vi "get_spiral_parameters.vi"(8 "error in (no error)":errorcluster, 11 "ImageAssemblerRK110612Spiral in":refnum<class "ImageAssemblerRK110612Spiral.lvclass">) -> (0 "error out":errorcluster, 2 "Fiber spiral parameters":T1={"Fiber Frequency"=2200, "Imaging Periods"=100, "Settling Periods"=50, "Resting Periods"=30, "Amplitude X"=0.5, "Amplitude Y"=0.5, "Phase difference"=90.0, "Initial Amplitude X"=0.0, "Initial Amplitude Y"=0.0} {"Initial Amplitude Y" min=0.0 max=3.0 step=0.1; "Initial Amplitude X" min=0.0 max=3.0 step=0.1; "Phase difference" min=0.0 max=360.0 step=5.0; "Amplitude Y" min=0.0 max=3.0 step=0.1; "Amplitude X" min=0.0 max=3.0 step=0.1}, 3 "ImageAssemblerRK110612Spiral out":refnum<class "ImageAssemblerRK110612Spiral.lvclass">)   [LabVIEW 2010, in "ImageAssemblerRK110612Spiral.lvclass"]
uses:
  ImageAssemblerRK110612Spiral.lvclass
  FPGAWrapper/FPGAWrapperRK110512Fiber/FPGAWrapperRK110512Fiber_Spiral/fiber_spiral_parameters.ctl
  ImageAssemblerRK110612Spiral.lvclass/ImageAssemblerRK110612Spiral.ctl
  FPGAWrapper/FPGAWrapperRK110512Fiber/FPGAWrapperRK110512Fiber_Spiral/FPGAWrapperRK110512Fiber_Spiral.lvclass
panel:
  # "[Hz]"
  # "[V]"
  # "[V]"
  # "[deg]"
  # "[V]"
  # "[V]"
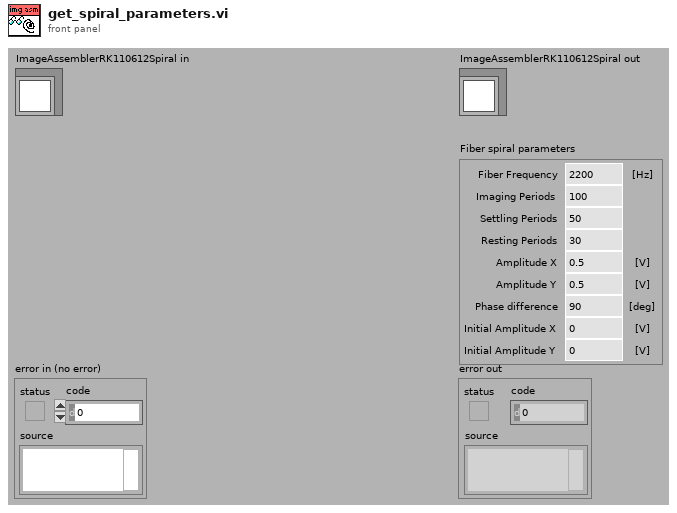
[diagram p1: front panel]
types:
  T1 = typedef "FPGAWrapperRK110512Fiber_Spiral.lvclass/fiber_spiral_parameters.ctl" = cluster{"Fiber Frequency":u16, "Imaging Periods":u16, "Settling Periods":u16, "Resting Periods":u16, "Amplitude X":dbl, "Amplitude Y":dbl, "Phase difference":dbl, "Initial Amplitude X":dbl, "Initial Amplitude Y":dbl}
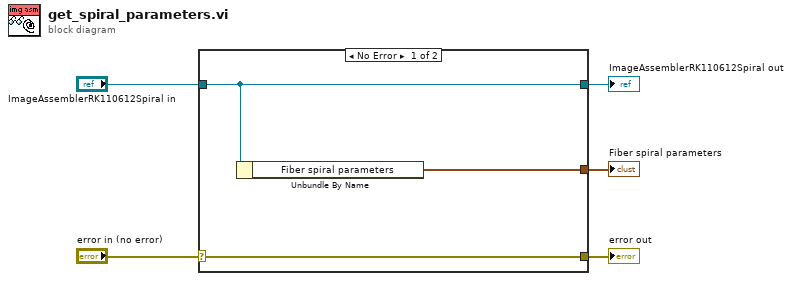
[diagram p0: block diagram]
diagram:
  n1 = case shown="No Error" "error in (no error)" {
    selector: "error in (no error)" -> [w8 w9]
    tunnel: [w8 w9] -> w4
    tunnel: [w7 w10] -> w2
    tunnel: "ImageAssemblerRK110612Spiral in" -> [w7 w10]
    tunnel: [w6 _] -> w1
    frame No Error {
      n2 = Unbundle By Name(w7) -> ("Fiber spiral parameters"=w6:T1)
    }
    frame Error {
    }
  }
  "error out" <- w4
  "ImageAssemblerRK110612Spiral out" <- w2
  "Fiber spiral parameters" <- w1
